vi "dashboard.vi"(11 "Array - String":string[](array[string])) -> (0 "total":i32, 1 "not available":i32, 2 "hardcopy":i32, 3 "softcopy":i32)   [LabVIEW 2018]
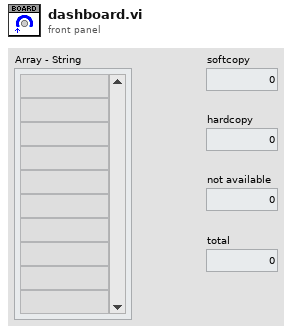
[diagram p1: front panel]
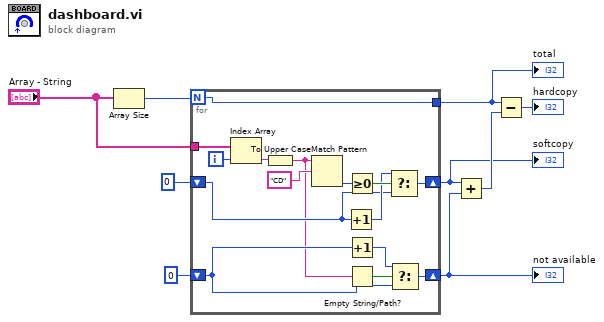
[diagram p0: block diagram]
diagram:
  n1 = Array Size(array="Array - String") -> (size(s)=w9:i32)
  n2 = for {
    N: w9 -> [w12]
    tunnel: "Array - String" -> [w24]
    shift-right: [w18] -> w2
    shift-left: 0 -> [w16]
    shift-right: [w15] -> w5
    shift-left: 0 -> [w14]
    tunnel: [w12] -> w1
    i -> [w23]
    n3 = Index Array(array=w24, index=w23) -> (element=w11:string)
    n4 = To Upper Case(1:w11) -> (0:w10:string)
    n5 = Match Pattern(string=w10, regular expression="CD") -> (offset past match=w21:i32)  [unwired: 1 in, 3 out]
    n6 = Increment(x=w16) -> (x+1=w19:i32)
    n7 = Greater Or Equal To 0?(x=w21) -> (x >= 0?=w20:bool)
    n8 = Increment(x=w14) -> (x+1=w13:i32)
    n9 = Empty String/Path?(string/path=w10) -> (empty?=w17:bool)
    n10 = Select(t=w19, s=w20, f=w16) -> (s? t:f=w18:i32)
    n11 = Select(t=w13, s=w17, f=w14) -> (s? t:f=w15:i32)
  }
  "softcopy" <- w2
  "not available" <- w5
  "total" <- w1
  n12 = Add(x=w2, y=w5) -> (x+y=w4:i32)
  n13 = Subtract(x=w1, y=w4) -> (x-y=→"hardcopy":i32)
